vi "BotSpeak_AnalogIn.vi"(2 "Bot Settings":T1, 3 "A/D Channel":u8(slide) scale=0.0..10.0) -> (1 "voltage":dbl(knob) scale=-10.0..10.0, 4 "Bot Settings":T1)   [LabVIEW 2012]
doc: "Reads and outputs the \"voltage\" into the specified \"A/D Channel\"."
uses:
  <userlib>/BotSpeak/VIs/Direct/BotSpeak_Control.ctl
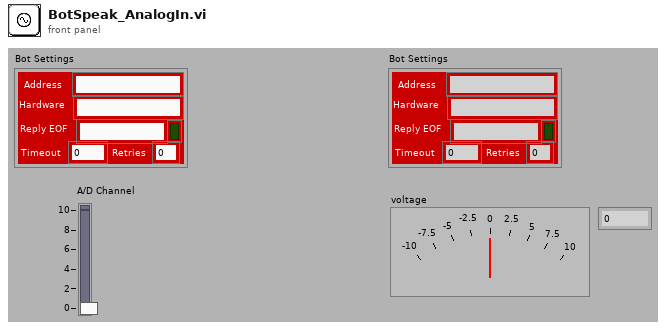
[diagram p1: front panel]
types:
  T1 = typedef "BotSpeak_Control.ctl" = cluster{"Address":string, "Reply EOF":string, "Hardware":string, "Retries":i8, "Timeout":i32, "Open?":bool}
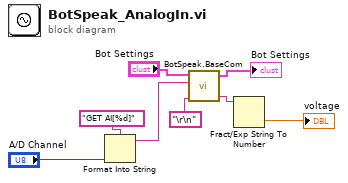
[diagram p0: block diagram]
diagram:
  n1 = Format Into String(format string="GET AI[%d]" ("command"), "A/D Channel") -> (resulting string=w8:string)  [unwired: 2 in, 1 out]
  n2 = call <userlib>:"BotSpeak.BaseCom.vi"("Termination"="\r\n", "command"=w8, "Bot Settings in"="Bot Settings") -> ("response"=w4:string, "Bot Settings out"=→"Bot Settings":T1)  [unwired: 2 in]
  n3 = Fract/Exp String To Number(string=w4) -> (number=→"voltage":dbl)  [unwired: 3 in, 1 out]
